vi "Constant getImage.vi"(1 "Image Index":enum16{"Acromass Logo"}(ring)) -> (0 "element":T1)   [LabVIEW 2018]
uses:
  <vilib>/picture/picture.llb/imagedata.ctl
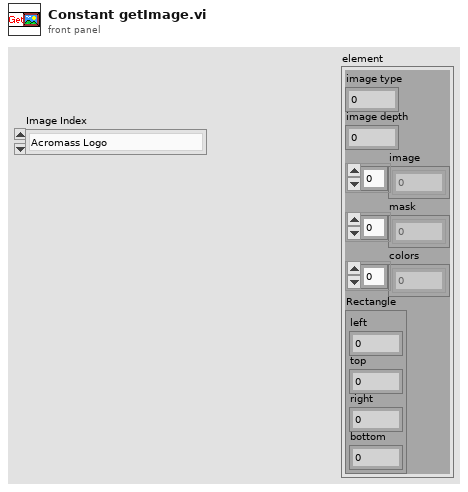
[diagram p1: front panel]
types:
  T1 = typedef "imagedata.ctl" = cluster{"image type":i32, "image depth":i32, "image":u8[], "mask":u8[], "colors":u32[], "Rectangle":cluster{"left":i16, "top":i16, "right":i16, "bottom":i16}}
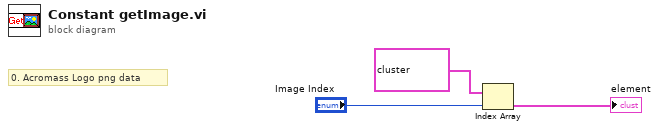
[diagram p0: block diagram]
diagram:
  # "0. Acromass Logo png data"
  n1 = Index Array(array=T1[] [{"image type"=0, "image depth"=32, "image"=array[124320 elements], "mask"=array[3996 elements], "colors"=[], "Rectangle"={"left"=0, "top"=0, "right"=280, "bottom"=111}}], index="Image Index") -> (element=→"element":T1)
